vi "new path.vi"(9 "Origin and Axis path":path, 10 "position path":path, 11 "controller":T1) -> (3 "controller 2":T1)   [LabVIEW 2016]
uses:
  Classes/Controller/Motion/A3200 Folder/A3200.lvclass
  Classes/Controller/Dispenser/Ultimus V2 Folder/Ultimus V2.lvclass
  Classes/Controller/I-O/NI-DAQ Folder/NI-DAQ.lvclass
  Classes/Controller/Motion/Motion Folder/Motion.lvclass
  Classes/Controller/I-O/I-O Folder/I-O.lvclass
  Classes/Controller/Dispenser/Dispenser Folder/Dispenser.lvclass
  <vilib>/Utility/file.llb/Read Delimited Spreadsheet (DBL).vi
panel:
  in  "add new position":bool
  in  "stop":bool
  in  "Tab Control":enum32{"Page 1", "controller"}(tab)
  out "read data":dbl[][](array[numeric])
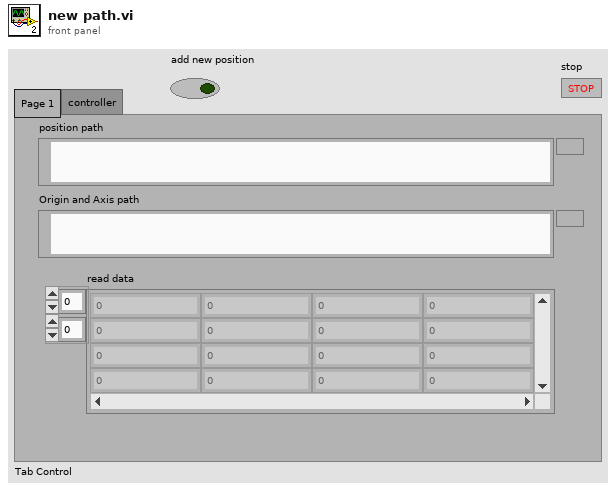
[diagram p1: front panel]
types:
  T1 = cluster{"A3200.lvclass":refnum<class "A3200.lvclass">, "Ultimus V2.lvclass":refnum<class "Ultimus V2.lvclass">, "NI-DAQ.lvclass":refnum<class "NI-DAQ.lvclass">, "Motion.lvclass":refnum<class "Motion.lvclass">, "I-O.lvclass":refnum<class "I-O.lvclass">, "Dispenser.lvclass":refnum<class "Dispenser.lvclass">}
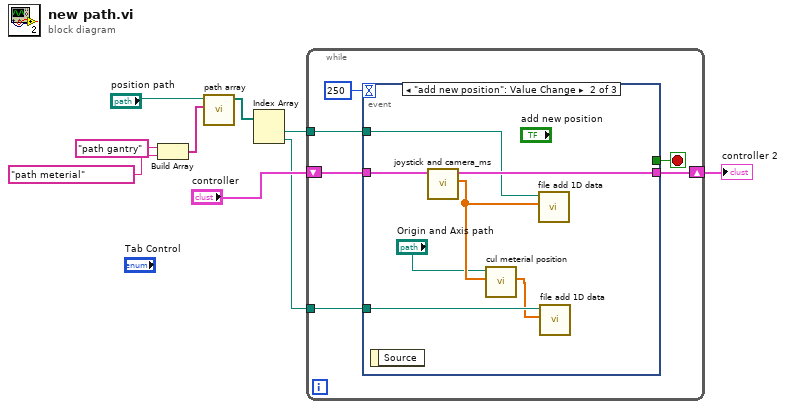
[diagram p0: block diagram]
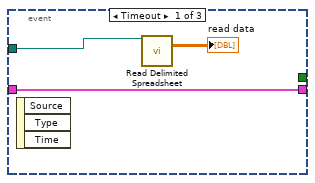
[diagram p2: hidden frame]
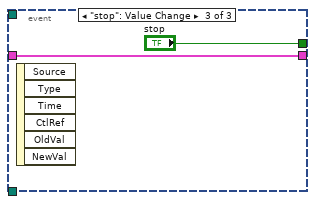
[diagram p3: hidden frame]
diagram:
  n1 = Build Array("path gantry", "path meterial") -> (w3:string[])
  n2 = call "path array.vi"("Array"=w3, "file path (dialog if empty)"="position path") -> ("path array"=w7:path[])  [unwired: 9 in]
  n3 = Index Array(array=w7) -> (element #1=w2:path, element #2=w1:path)  [unwired: 2 in]
  n4 = while {
    shift-right: [w12] -> w8
    shift-left: "controller" -> [w13]
    tunnel: w2 -> [w11]
    tunnel: w1 -> [w10]
    stop <- w15 stop-if-true
    n5 = event shown="[1] \"add new position\": Value Change" {
      selector: _ -> [_ _ _]
      dyn-events: _ -> [_ _ _]
      timeout: 250 -> [_ _ _]
      tunnel: [_ _ "stop"] -> w15
      tunnel: w11 -> [w18 w23 _]
      tunnel: w13 -> [w17 w25 w26]
      tunnel: [w17 w24 w26] -> w12
      tunnel: w10 -> [_ w22 _]
      event Timeout {
        n6 = event-data() -> ()  [unwired: 1 in, 3 out]
        n7 = call-poly <vilib>:"Read Delimited Spreadsheet.vi"("file path (dialog if empty)"=w18) -> ("all rows"=→"read data":dbl[][])  [unwired: 9 in, 5 out]
      }
      event "add new position": Value Change {
        n8 = event-data() -> ()  [unwired: 1 in, 1 out]
        n9 = call "joystick and camera_ms.vi"("controller in"=w25) -> ("Gantry"=w20:dbl[], "controller out"=w24:T1)  [unwired: 9 in]
        n10 = call "cul meterial position.vi"("position in"=w20, "Origin and Axis path"="Origin and Axis path") -> ("position out"=w21:dbl[])  [unwired: 9 in]
        n11 = call "file add 1D data.vi"("element"=w20, "file path (dialog if empty)"=w23) -> ()  [unwired: 10 in]
        n12 = call "file add 1D data.vi"("element"=w21, "file path (dialog if empty)"=w22) -> ()  [unwired: 10 in]
      }
      event "stop": Value Change {
        n13 = event-data() -> ()  [unwired: 1 in, 6 out]
      }
    }
  }
  "controller 2" <- w8
